vi "resetOutputPressure.vi"(8 "error in (no error)":errorcluster, 11 "Model in":refnum<class "Model.lvclass">) -> (0 "error out":errorcluster, 3 "Model out":refnum<class "Model.lvclass">)   [LabVIEW 2015, in "Model.lvclass"]
uses:
  Model.lvclass
  Model.lvclass/Model.ctl
  <userlib>/Common/Devices/PressureValve/PressureValve/PressureValve.lvclass/PressureValve.ctl
  <userlib>/Common/Devices/PressureValve/PressureValve/PressureValve.lvclass
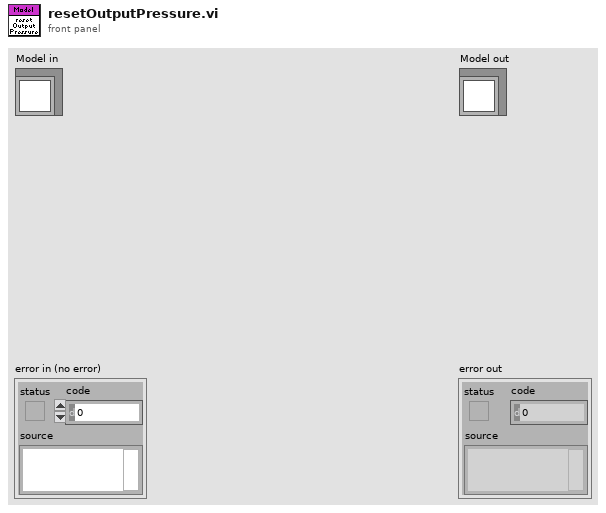
[diagram p1: front panel]
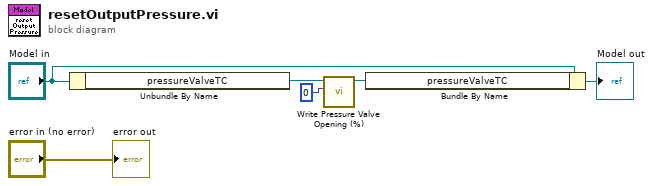
[diagram p0: block diagram]
diagram:
  n1 = Unbundle By Name("Model in") -> ("pressureValveTC"=w5:refnum<class "PressureValveTC.lvclass">)
  n2 = call <userlib>:"Write Pressure Valve Opening (%).vi"("Pressure Valve Opening (%)"=u16 0 ("Ramp Output"), "PressureValve in"=w5) -> ("PressureValve out"=w4:refnum<class "PressureValveTC.lvclass">)  [unwired: 9 in]
  n3 = Bundle By Name(cluster="Model in", "pressureValveTC"=w4) -> (→"Model out":refnum<class "Model.lvclass">)
  "error out" <- "error in (no error)"
